vi "CRYHanning Correction.vi"(2 "window":u16, 4 "N sine":i32, 5 "N FFT":i32, 6 "frequency":dbl, 7 "Fs":i32) -> (0 "Complex correction factor":cdb format="%.2f", 1 "Index sine":i32)   [LabVIEW 2013]
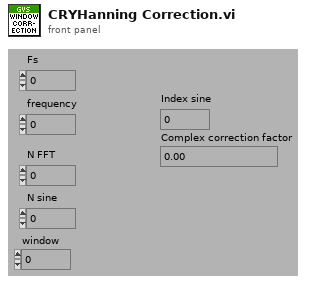
[diagram p1: front panel]
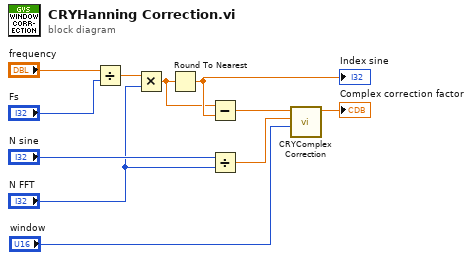
[diagram p0: block diagram]
diagram:
  n1 = Divide(x="frequency", y="Fs") -> (x/y=w9:dbl)
  n2 = Multiply(x=w9, y="N FFT") -> (x*y=w4:dbl)
  n3 = Round To Nearest(number=w4) -> (nearest integer value=w8:dbl)
  "Index sine" <- w8
  n4 = Subtract(x=w4, y=w8) -> (x-y=w2:dbl)
  n5 = Divide(x="N sine", y="N FFT") -> (x/y=w3:dbl)
  n6 = call "CRYComplex Correction.vi"("window"="window", "Beta(relative record after zero pad.:0.5..1.0"=w3, "Alpha(dev. from line freq.: -0.5..0.5 delta f)"=w2) -> ("Complex correction factor"=→"Complex correction factor":cdb)  [unwired: 6 in]
